vi "PI Ask for Communication Parameters.vi"() -> (10 "Termination character out":T2[](array[typedef])=[enum."LF"], 11 "Syntax out":T1[](array[typedef])=[enum."GCS 1.0"], 12 "TCP/IP Configuration out":T3(array[cluster])=[{"Host address/name"="localhost", "Port"=50000, "Board"=0}], 13 "Flow control out":T6(array[cluster])=[{"input XON/XOFF"=FALSE, "input HW Handshake"=FALSE, "input alt HW HShk"=FALSE, "output XON/XOFF"=FALSE, "output HW Handshake"=FALSE, "output alt HW HShk"=FALSE, "XOFF byte "=19, "XON byte"=17, "parity error byte"=0}] {"parity error byte" format="%.0x"; "XON byte" format="%.0x"; "XOFF byte" format="%.0x"}, 15 "How many\nsystems? out":i32=1 min=1 max=4 step=1, 16 "Abort out":bool=TRUE, 17 "Interface configuration out":T14(array[cluster])=[{"RS232 Portnumber"=0, "Timeout"=1000, "RS232 baud rate"=57600, "Interface"=0, "GPIB Bus"=0, "GPIB address"=4, "GPIB Mode"=0}] {"Interface" items=["RS232", "GPIB", "DLL", "TCP-IP", "USB", "Analog"]; "RS232 Portnumber" items=["COM1", "COM2", "COM3", "COM4", "COM5", "COM6", "COM7", "COM8", "COM9", "COM10", "COM11", "COM12", "COM13", "COM14", "COM15", "COM16", "COM17", "COM18", "COM19", "COM20", "COM21", "COM22", "COM23", "COM24", "COM25", "COM26", "COM27", "COM28", "COM29", "COM30"]}, 18 "DLL Interface\nconfiguration out":T11(array[cluster])=[{"DLL for Device"=0, "DLL Interface"=2, "Parameter"="1"}] {"DLL for Device" items=["C-843", "C-844", "E-710", "C-843.PM", "C-865", "E-761", "Mercury", "E-755", "E-753", "C-866", "E-712", "E-725", "E-861", "C-867", "E-517", "E-816", "E-709", "PI_GCS2_DLL", "HydraPollux"]; "DLL Interface" items=["RS232", "GPIB", "Board", "TCP-IP", "USB", "RS232_DC", "USB_DC", "TCPIP_DC"]})   [LabVIEW 2020]
doc: "A user-interface VI for setting up communications parameters (RS-232 or GPIB, number of systems, baudrate, timeout etc.) for up to 4 systems. Press F1 for displaying a help window with the appropriate interface configuration of each PI controller."
uses:
  Available interfaces.ctl
  Available DLLs.ctl
  Available DLL interfaces.ctl
  Termination character.ctl
  Syntax.ctl
panel:
  in  "Hide help":bool
  in  "Show help":bool
  in  "Help string":string="\nHELP for PI Ask for Communication Parameters.vi\n\nThis VI is a user-interface VI for setting up communications parameters (interface type, number of systems, baudrate, timeout etc.) for up to 4 systems.\nSelect the number of connected systems first. Select the corresponding interface configuration parameters then in the order described below.\n\nPress F10 to return to the VI.\n\nC-413: \tInterface = RS232, DLL, or TCP/IP. TCP/IP support available depending on controller version! If unsure whether your controller supports TCP/IP communication, please refer to the controller user manual), RS232: Input and output HW handshake must be TRUE. DLL: DLL for Device = PI_GCS2_DLL, DLL Interface = USB, Parameter = Serial no. of system to connect to. Syntax: GCS 2.0; Term char = LF.\n\nC-414: \tInterface = RS232, DLL, or TCP/IP. RS232: Input and output HW handshake must be TRUE. DLL: DLL for Device = PI_GCS2_DLL, DLL Interface = USB, Parameter = Serial no. of system to connect to. Syntax: GCS 2.0; Term char = LF.\n\nC-702: \tInterface = RS232 or TCP/IP, RS232: Input and output HW handshake \tmust \tbe TRUE. Syntax: GCS 1.0; Term char = LF.\n\nC-843: \tInterface = DLL, DLL for Device = C-843, DLL Interface = Board, \tParameter = Board number (1 for first C-843 board). Syntax: GCS 1.0; \tTerm char = LF.\n\nC-843.PM: \tInterface = DLL, DLL for Device = C-843.PM, DLL Interface = Board, \tParameter = Board number (1 for first C-843 board). Syntax: GCS 1.0; \tTerm char = LF.\n\nC-865: \tInterface = DLL, DLL for Device = C-865, DLL Interface = RS232, \tParameter = empty string, RS232 baud rate = set as appropriate. Syntax: \tGCS 1.0; Term char = LF.\n\nC-866: \tInterface = DLL, DLL for Device = C-866, DLL Interface = RS232 or USB, \tRS232: Parameter = empty string, RS232 baud rate = set as appropriate, \tUSB: Parameter = Serial no. of system to connect to, \n\tSyntax: GCS 1.0; Term char = LF.\n\nC-867: \tSingle Device: Interface = RS232, TCP/IP or DLL, RS232: Input and output HW \thandshake must be FALSE. DLL (USB): DLL for Device = C-867, DLL \tInterface = USB, Parameter = Serial no. of system to connect to.\nDaisyChain: Interface = DLL, DLL for Device = C-867, DLL Interface = \tRS232_DC, Parameter = Number of device in chain, \tRegister DC: \tFALSE. Syntax: GCS 2.0; Term char = LF.\n\nC-880, C-848: \tInterface = RS232 or GPIB, RS232: Input and output HW handshake must \tbe TRUE. Syntax: GCS 1.0; Term char = LF.\n\nC-880K005: \tInterface = RS232, Input and output HW handshake must be FALSE. \tSyntax: GCS 1.0; Term char = LF.\n\nC-884: \tInterface = RS232, TCP/IP or DLL, RS232: Input and output HW handshake must be FALSE. DLL (USB): DLL for Device = PI_GCS2_DLL, DLL Interface = USB, Parameter = Serial no. of system to connect to. Syntax: GCS 2.0; Term char = LF.\n\nC-885: \tInterface = TCP/IP or DLL. DLL (USB): DLL for Device = PI_GCS2_DLL, DLL Interface = USB, Parameter = Serial no. of system to connect to. Syntax: GCS 2.0; Term char = LF.\nDaisyChain: Interface = DLL, DLL for Device = PI_GCS2_DLL, DLL Interface = \tTCPIP_DC or USB_DC, Parameter = Number of device in chain, \tRegister DC: \tFALSE. Syntax: GCS 2.0; Term char = LF.\n\nC-886: \tInterface = TCP/IP or DLL. DLL (USB): DLL for Device = PI_GCS2_DLL, DLL Interface = USB, Parameter = Serial no. of system to connect to. Syntax: GCS 2.0; Term char = LF.\n\nC-887, F-206, M-8X0: \tFor GCS syntax version = GCS 1.0 (older firmware or compatibility mode, \tcan be set with CSV.vi), Interface = RS232, GPIB (not available for C-887 \tcontroller) or TCP/IP., The error status will not be cleared by this VI. The \tfirst ERR? query will report a hidden error with error code 1, which will be \tcleared during system initialization (INI). RS232: Input and output \thandshake settings must be FALSE. Syntax: GCS 1.0; Term char = \tLF.\nFor GCS syntax version = GCS 2.0 (C-887 Controller), Interface = RS232 \tor TCP/IP. RS232: Input and output handshake settings must be FALSE. \tSyntax: GCS 2.0; Term char = LF.\n\nE-135: Interface = RS232, TCP/IP or DLL: Input and output HW \thandshake must be FALSE. DLL (USB): DLL for Device = \tPI_GCS2_DLL, DLL Interface = USB, Parameter = Serial no. of system to \tconnect to. Syntax: GCS 2.0; Term char = LF.\n\nE-516: \tInterface = RS232 or GPIB, RS232: Input and output HW handshake must \tbe TRUE. Syntax: GCS 1.0; Term char = LF.\n\nE-517: \tInterface = RS232, GPIB, TCP/IP or DLL, RS232: Input and output HW \thandshake must be TRUE, DLL (USB): DLL for Device = E-517, DLL \tInterface = USB, Parameter = Serial no. of system to connect to. Syntax: GCS 2.0; Term char = LF.\n\nE-518: \t\tInterface = RS232, TCP/IP or DLL, RS232: Input and output HW handshake must be TRUE, DLL (USB): DLL for Device = PI_GCS2_DLL, DLL Interface = USB, Parameter = Serial no. of system to connect to. Syntax: GCS 2.0; Term char = LF.\n\nE-709: \tInterface = RS232 or DLL, RS232: Input and output HW handshake \tmust be TRUE. DLL (USB): DLL for Device = E-709, DLL Interface = USB, \tParameter = Serial no. of system to connect to. Syntax: GCS 2.0; Term \tchar = LF.\n\nE-710:\tInterface = DLL, DLL for Device = E-710, DLL Interface = RS232 or GPIB, \tParameter = empty string. Syntax: GCS 1.0; Term char = LF.\n\nE-712: \tInterface = RS232, TCP/IP or DLL, RS232: Input and output HW \thandshake must be TRUE. DLL: DLL for Device = E-712, DLL Interface = \tUSB, \tParameter = Serial no. of system to connect to. \n\tSyntax: GCS 2.0; Term char = LF.\n\nE-725: \tInterface = RS232, TCP/IP or DLL, RS232: Input and output HW \thandshake must be TRUE. DLL: DLL for Device = E-725, DLL Interface = \tUSB, \tParameter = Serial no. of system to connect to. \nSyntax: GCS 2.0; Term char = LF.\n\nE-727: \tInterface = RS232, TCP/IP or DLL, RS232: Input and output HW \thandshake must be TRUE. DLL: DLL for Device = PI_GCS2_DLL, DLL Interface = \tUSB, \tParameter = Serial no. of system to connect to. Syntax: GCS 2.0; Term char = LF.\n\nE-753: \tInterface = RS232 or TCP/IP, RS232: Input and output HW handshake \tmust \tbe TRUE. Syntax: GCS 2.0; Term char = LF.\n\nE-754: Interface = RS232, TCP/IP or DLL, RS232: Input and output HW handshake must be TRUE. DLL: DLL for Device = E-754, DLL Interface = USB, Parameter = Serial no. of system to connect to. Syntax: GCS 2.0; Term char = LF.\n\nE-755:\tSingle Device: Interface = RS232, Input and output HW handshake must \tbe TRUE. DaisyChain: Interface = DLL, DLL for Device = E-755, DLL \tInterface = RS232_DC, Parameter = Number of device in chain (first \tdevice: 1). Syntax: GCS 2.0; Term char = LF.\n\nE-761:\tInterface = DLL, DLL for Device = E-761, DLL Interface = Board, \tParameter = Board number (1 for first E-761 board). Syntax: GCS 1.0; \tTerm char = LF.\n\nE-816: \tInterface = RS232 or DLL, RS232: Input and output HW handshake must \tbe TRUE. DLL (USB): DLL for Device = E-816, DLL Interface = USB, \tParameter = Serial no. of system to connect to. Syntax: GCS 1.0; Term \tchar = LF. \n\nE-861: \tSingle Device: Interface = RS232 or DLL, RS232: Input and output HW \thandshake must be FALSE. DLL (USB): DLL for Device = E-861, DLL \tInterface = USB, Parameter = Serial no. of system to connect to.\nDaisyChain: Interface = DLL, DLL for Device = E-861, DLL Interface = \tRS232_DC or USB_DC, Parameter = Number of device in chain (first device: 1), \tRegister DC: FALSE. Syntax: GCS 2.0; Term char = LF.\n\nE-870: \tInterface = DLL, DLL (USB): DLL for Device = PI_GCS2_DLL, DLL \tInterface = USB, Parameter = Serial no. of system to connect to.\nSyntax: GCS 2.0; Term char = LF.\n\nE-871: Single Device: Interface = RS232 or DLL, RS232: Input and output HW \thandshake must be FALSE. DLL (USB): DLL for Device = \tPI_GCS2_DLL, DLL Interface = USB, Parameter = Serial no. of system to \tconnect to.\nDaisyChain: Interface = DLL, DLL for Device = PI_GCS2_DLL, DLL \tInterface = RS232_DC or USB_DC, Parameter = Number of device in \tchain, Register DC: FALSE. Syntax: GCS 2.0; Term char = LF.\n\nE-872: Interface = RS232, TCP/IP or DLL, RS232: Input and output HW handshake must be FALSE. DLL (USB): DLL for Device = PI_GCS2_DLL, DLL Interface = USB, Parameter = Serial no. of system to \tconnect to.\n\nE-873: Interface = RS232, TCP/IP or DLL, RS232: Input and output HW handshake must be FALSE. DLL (USB): DLL for Device = PI_GCS2_DLL, DLL Interface = USB, Parameter = Serial no. of system to \tconnect to.\n\nE-874: Interface = RS232, TCP/IP or DLL, RS232: Input and output HW handshake must be FALSE. DLL (USB): DLL for Device = PI_GCS2_DLL, DLL Interface = USB, Parameter = Serial no. of system to \tconnect to\n\nHydra: \tInterface = DLL, DLL (TCP/IP and RS-232): DLL for Device = \t\tPI_HydraPollux_GCS2_DLL, DLL Interface = RS232 or TCP/IP, Syntax: \tGCS 2.0; Term char = LF.\n\nMercury™: \tInterface = DLL, DLL for Device = Mercury™, DLL Interface = RS232 \t(even if using USB), Parameter = empty string, RS232 baud rate = same \tas set on controller hardware, Syntax: GCS 1.0; Term char = LF.\n\nGCS_Mercury: \tSingle Device: Interface = RS232 or DLL, RS232: Input and output HW \thandshake must be FALSE. DLL (USB): DLL for Device = PI_GCS2_DLL, \tDLL Interface = USB, Parameter = Serial no. of system to connect to. \tDaisyChain: Interface = DLL, DLL for Device = PI_GCS2_DLL, DLL \tInterface = RS232_DC or USB_DaisyChain, Parameter = Number of device in chain, \tRegister DC: \tFALSE. Syntax: GCS 2.0; Term char = LF.\n\nPollux: \tInterface = DLL, DLL (RS-232): DLL for Device = PI_HydraPollux_GCS2_DLL, DLL Interface = RS232, Baudrate must be 19200, Syntax: GCS 2.0; Term char = LF.\n\n"
  in  "TCP/IP\nConfiguration 2":T4={"Host address/name"="Z-A521-2.pi.ws", "Port"=3000, "Board"=0}
  in  "RS 16":string
  in  "RS 15":string
  in  "RS 14":string
  in  "RS 13":string
  in  "Flow control":T5={"input XON/XOFF"=FALSE, "input HW Handshake"=FALSE, "input alt HW HShk"=FALSE, "output XON/XOFF"=FALSE, "output HW Handshake"=FALSE, "output alt HW HShk"=FALSE, "XOFF byte "=19, "XON byte"=17, "parity error byte"=0} {"parity error byte" format="%.0x"; "XON byte" format="%.0x"; "XOFF byte" format="%.0x"}
  in  "RS 12":string
  in  "RS 11":string
  in  "RS 10":string
  in  "RS 9":string
  in  "RS 8":string
  in  "RS 7":string
  in  "RS 6":string
  in  "RS 5":string
  in  "RS 4":string
  in  "RS 3":string
  in  "RS 2":string
  in  "RS1":string
  in  "DLL Interface\nConfiguration 2":T7 {"DLL Interface" items=["RS232", "GPIB", "Board"]; "DLL for Device" items=["C-843", "C-844"]}
  in  "Interface configuration 2":T8={"RS232 Portnumber"=0, "Timeout"=5000, "RS232 Baud rate"=56000, "Interface"=0, "GPIB Bus"=0, "GPIB Address"=4, "GPIB Mode"=0} {"Interface" items=["RS232", "GPIB", "DLL"]; "RS232 Portnumber" items=["COM1", "COM2", "COM3", "COM4", "COM5", "COM6", "COM7", "COM8", "COM9"]}
  in  "String4":string="System No. 4"
  in  "String3":string="System No. 3"
  in  "String2":string="System No. 2"
  in  "String1":string="System No. 1"
  in  "Interface configuration":T13(array[cluster])=[{"RS232 Portnumber"=0, "Timeout"=1000, "GPIB Bus"=0, "GPIB Address"=4, "GPIB Mode"=0, "DLL for Device"=17, "DLL Interface"=4, "Parameter"="1", "Handshake"=0, "Interface"=0, "Termchar"=enum."LF", "Host address/name"="localhost", "Port"=50000, "Board"=0, "RS232 Baud rate"=4, "Syntax"=enum."GCS 2.0"}, {"RS232 Portnumber"=0, "Timeout"=1000, "GPIB Bus"=0, "GPIB Address"=4, "GPIB Mode"=0, "DLL for Device"=0, "DLL Interface"=2, "Parameter"="1", "Handshake"=0, "Interface"=3, "Termchar"=enum."LF", "Host address/name"="localhost", "Port"=50000, "Board"=0, "RS232 Baud rate"=4, "Syntax"=enum."GCS 1.0"}, {"RS232 Portnumber"=0, "Timeout"=1000, "GPIB Bus"=0, "GPIB Address"=4, "GPIB Mode"=0, "DLL for Device"=0, "DLL Interface"=2, "Parameter"="1", "Handshake"=0, "Interface"=1, "Termchar"=enum."LF", "Host address/name"="localhost", "Port"=50000, "Board"=0, "RS232 Baud rate"=4, "Syntax"=enum."GCS 1.0"}, {"RS232 Portnumber"=0, "Timeout"=1000, "GPIB Bus"=0, "GPIB Address"=4, "GPIB Mode"=0, "DLL for Device"=0, "DLL Interface"=2, "Parameter"="1", "Handshake"=0, "Interface"=2, "Termchar"=enum."LF", "Host address/name"="localhost", "Port"=50000, "Board"=0, "RS232 Baud rate"=4, "Syntax"=enum."GCS 1.0"}] {"RS232 Baud rate" items=["9600", "14400", "19200", "38400", "57600", "115200"]; "Interface" items=["RS232", "GPIB", "DLL", "TCP-IP", "USB", "Analog"]; "Handshake" items=["None", "HW", "XON/XOFF"]; "DLL Interface" items=["RS232", "GPIB", "Board", "TCP-IP", "USB", "RS232_DC", "USB_DC", "TCPIP_DC"]; "DLL for Device" items=["C-843", "C-844", "E-710", "C-843.PM", "C-865", "E-761", "Mercury", "E-755", "E-753", "C-866", "E-712", "E-725", "E-861", "C-867", "E-517", "E-816", "E-709", "PI_GCS2_DLL", "HydraPollux"]; "RS232 Portnumber" items=["COM1", "COM2", "COM3", "COM4", "COM5", "COM6", "COM7", "COM8", "COM9", "COM10", "COM11", "COM12", "COM13", "COM14", "COM15", "COM16", "COM17", "COM18", "COM19", "COM20", "COM21", "COM22", "COM23", "COM24", "COM25", "COM26", "COM27", "COM28", "COM29", "COM30"]}
  in  "Number of systems":i32=1 min=1 max=4 step=1
  in  "abort":bool=TRUE
  in  "ok":bool
  # "Select Interface Parameters"
  # "Interface configuration"
  # "General:"
  # "RS232:"
  # "GPIB:"
  # "DLL:"
  # "TCP/IP:"
  # "TCP/IP:"
  # "TCP/IP:"
  # "DLL:"
  # "General:"
  # "RS232:"
  # "GPIB:"
  # "DLL:"
  # "General:"
  # "RS232:"
  # "GPIB:"
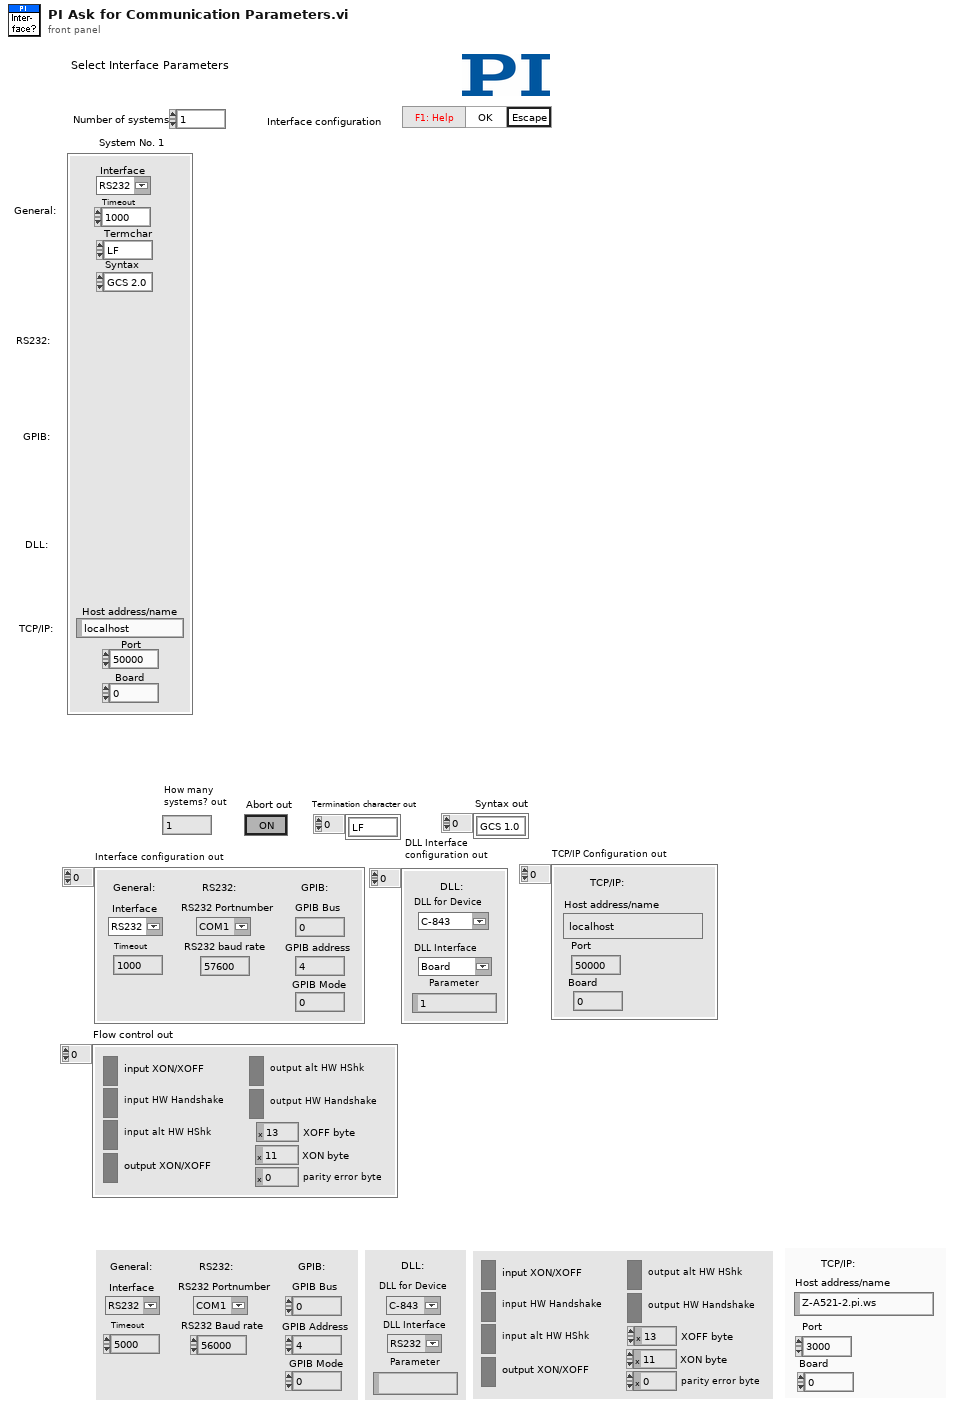
[diagram p1: front panel]
types:
  T1 = typedef "Syntax.ctl" = enum16{"GCS 1.0", "GCS 2.0", "GCS 3.0"}
  T2 = typedef "Termination character.ctl" = enum16{"LF", "CR", "LFCR", "CRLF"}
  T3 = cluster{"Host address/name":string, "Port":i32, "Board":i32}[]
  T4 = cluster{"Host address/name":string, "Port":i32, "Board":i32}
  T5 = cluster{"input XON/XOFF":bool, "input HW Handshake":bool, "input alt HW HShk":bool, "output XON/XOFF":bool, "output HW Handshake":bool, "output alt HW HShk":bool, "XOFF byte ":u8, "XON byte":u8, "parity error byte":u16}
  T6 = cluster{"input XON/XOFF":bool, "input HW Handshake":bool, "input alt HW HShk":bool, "output XON/XOFF":bool, "output HW Handshake":bool, "output alt HW HShk":bool, "XOFF byte ":u8, "XON byte":u8, "parity error byte":u16}[]
  T7 = cluster{"DLL for Device":u16, "DLL Interface":u16, "Parameter":string}
  T8 = cluster{"RS232 Portnumber":u16, "Timeout":u32, "RS232 Baud rate":u32, "Interface":u16, "GPIB Bus":i16, "GPIB Address":i16, "GPIB Mode":i16}
  T9 = typedef "Available DLLs.ctl" = u16
  T10 = typedef "Available DLL interfaces.ctl" = u16
  T11 = cluster{"DLL for Device":T9, "DLL Interface":T10, "Parameter":string}[]
  T12 = typedef "Available interfaces.ctl" = u16
  T13 = cluster{"RS232 Portnumber":u16, "Timeout":i32, "GPIB Bus":i16, "GPIB Address":i16, "GPIB Mode":i16, "DLL for Device":T9, "DLL Interface":T10, "Parameter":string, "Handshake":u16, "Interface":T12, "Termchar":T2, "Host address/name":string, "Port":i32, "Board":i32, "RS232 Baud rate":u16, "Syntax":T1}[]
  T14 = cluster{"RS232 Portnumber":u16, "Timeout":u32, "RS232 baud rate":u32, "Interface":T12, "GPIB Bus":i16, "GPIB address":i16, "GPIB Mode":i16}[]
  T15 = cluster{"input XON/XOFF":bool, "input HW Handshake":bool, "input alt HW HShk":bool, "output XON/XOFF":bool, "output HW Handshake":bool, "output alt HW HShk":bool, "XOFF byte":u8, "XON byte":u8, "parity error byte":u16}[]
  T16 = cluster{"DLL for Device":u16, "DLL Interface":u16, "Parameter":string}[]
  T17 = cluster{"RS232 Portnumber":u16, "Timeout":u32, "RS232 Baud rate":u32, "Interface":T12, "GPIB Bus":i16, "GPIB Address":i16, "GPIB Mode":i16}[]
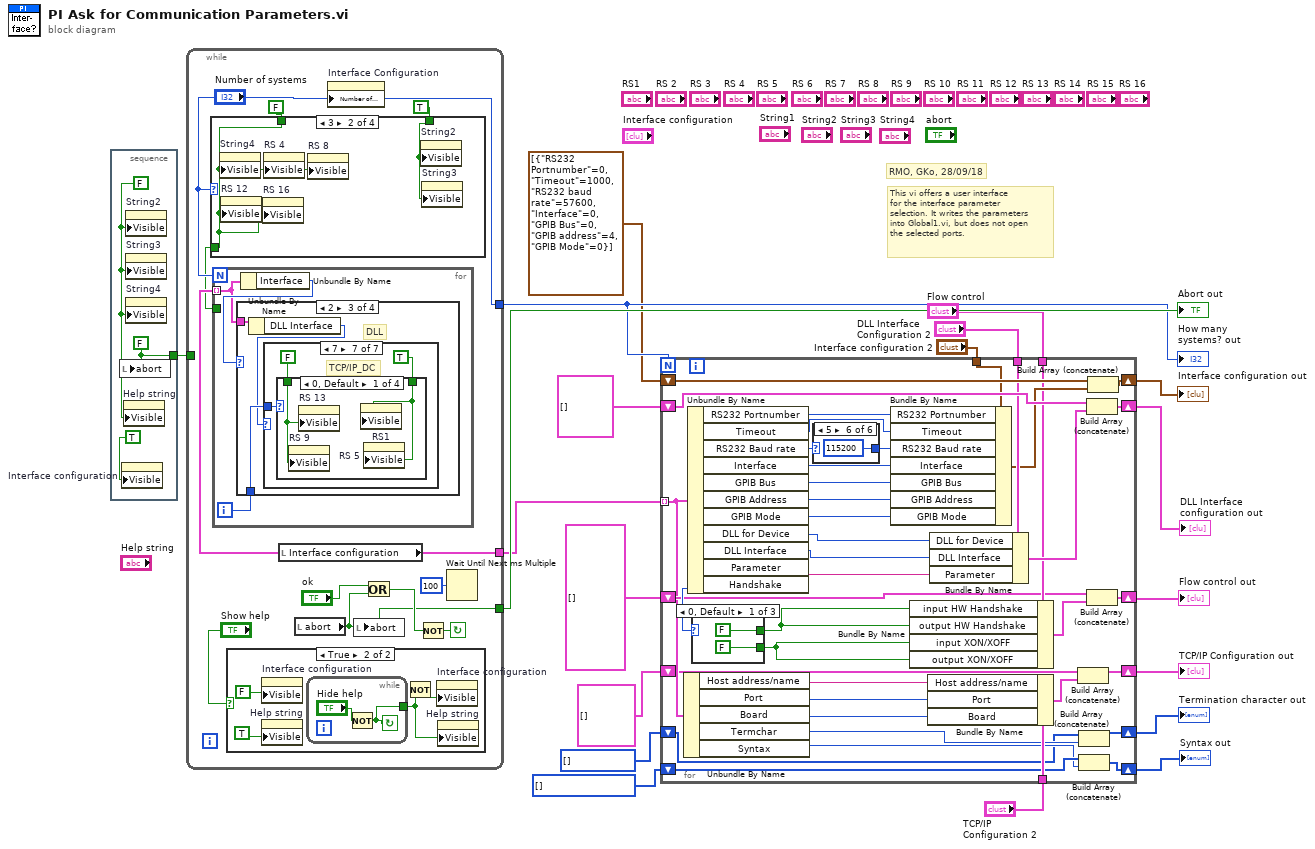
[diagram p0: block diagram]
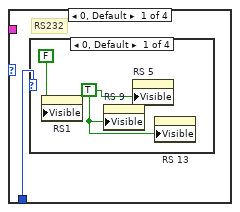
[diagram p3: hidden frame]
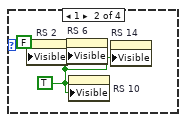
[diagram p4: hidden frame]
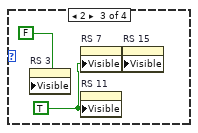
[diagram p5: hidden frame]
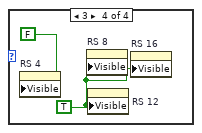
[diagram p6: hidden frame]
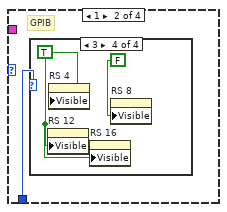
[diagram p7: hidden frame]
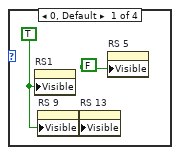
[diagram p8: hidden frame]
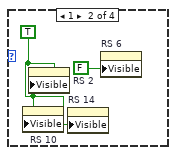
[diagram p9: hidden frame]
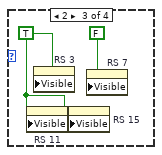
[diagram p10: hidden frame]
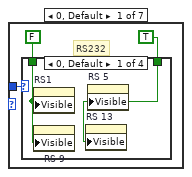
[diagram p11: hidden frame]
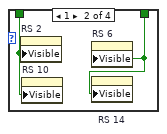
[diagram p12: hidden frame]
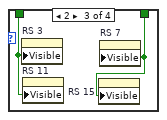
[diagram p13: hidden frame]
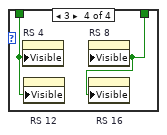
[diagram p14: hidden frame]
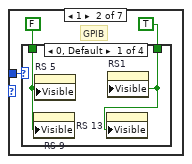
[diagram p15: hidden frame]
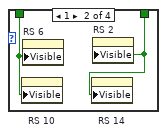
[diagram p16: hidden frame]
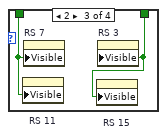
[diagram p17: hidden frame]
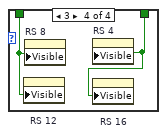
[diagram p18: hidden frame]
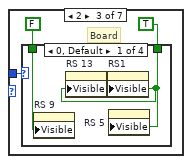
[diagram p19: hidden frame]
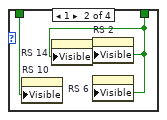
[diagram p20: hidden frame]
diagram:
  w2 = enum16{"GCS 1.0", "GCS 2.0"}[] [] items=["GCS 1.0", "GCS 2.0"]
  w5 = T2[] [] items=["LF", "CR", "LFCR", "CRLF"]
  # "This vi offers a user interface\nfor the interface parameter\nselection. It writes the parameters\ninto Global1.vi, but does not open\nthe selected ports."
  # "RMO, GKo, 28/09/18"
  n1 = stacked-sequence {
    tunnel: [w23] -> w12
    frame #0 {
      w22 = FALSE ("Write Attribute")
      w23 = FALSE
      n2 = local write "abort"(w23) -> ()
      n3 = property on="Interface configuration" class="Arr (strict)"("Visible"=TRUE) -> ()  [unwired: 2 in, 2 out]
      n4 = property on="Help string" class="Str"("Visible"=w22) -> ()  [unwired: 2 in, 2 out]
      n5 = property on="String2" class="Str"("Visible"=w22) -> ()  [unwired: 2 in, 2 out]
      n6 = property on="String3" class="Str"("Visible"=w22) -> ()  [unwired: 2 in, 2 out]
      n7 = property on="String4" class="Str"("Visible"=w22) -> ()  [unwired: 2 in, 2 out]
    }
  }
  n8 = while {
    tunnel: w12 -> [_]
    tunnel: ["Number of systems"] -> w19
    tunnel: [w31] -> w20
    tunnel: [w30] -> w15
    stop <- w33 continue-if-true
    n9 = case shown="3" "Number of systems" {
      tunnel: [w151 w153 w155 w156] -> w27
      tunnel: FALSE ("Write Attribute") -> [w151 w153 _ w156]
      tunnel: TRUE -> [w152 w154 w155 _]
      frame 2 {
        n10 = property on="String3" class="Str"("Visible"=w151) -> ()  [unwired: 2 in, 2 out]
        n11 = property on="String4" class="Str"("Visible"=w151) -> ()  [unwired: 2 in, 2 out]
        n12 = property on="RS 15" class="Str"("Visible"=w151) -> ()  [unwired: 2 in, 2 out]
        n13 = property on="RS 3" class="Str"("Visible"=w151) -> ()  [unwired: 2 in, 2 out]
        n14 = property on="RS 16" class="Str"("Visible"=w151) -> ()  [unwired: 2 in, 2 out]
        n15 = property on="RS 4" class="Str"("Visible"=w151) -> ()  [unwired: 2 in, 2 out]
        n16 = property on="RS 7" class="Str"("Visible"=w151) -> ()  [unwired: 2 in, 2 out]
        n17 = property on="RS 8" class="Str"("Visible"=w151) -> ()  [unwired: 2 in, 2 out]
        n18 = property on="RS 11" class="Str"("Visible"=w151) -> ()  [unwired: 2 in, 2 out]
        n19 = property on="RS 12" class="Str"("Visible"=w151) -> ()  [unwired: 2 in, 2 out]
        n20 = property on="String2" class="Str"("Visible"=w152) -> ()  [unwired: 2 in, 2 out]
      }
      frame 3 {
        n21 = property on="String4" class="Str"("Visible"=w153) -> ()  [unwired: 2 in, 2 out]
        n22 = property on="RS 12" class="Str"("Visible"=w153) -> ()  [unwired: 2 in, 2 out]
        n23 = property on="RS 16" class="Str"("Visible"=w153) -> ()  [unwired: 2 in, 2 out]
        n24 = property on="RS 4" class="Str"("Visible"=w153) -> ()  [unwired: 2 in, 2 out]
        n25 = property on="RS 8" class="Str"("Visible"=w153) -> ()  [unwired: 2 in, 2 out]
        n26 = property on="String2" class="Str"("Visible"=w154) -> ()  [unwired: 2 in, 2 out]
        n27 = property on="String3" class="Str"("Visible"=w154) -> ()  [unwired: 2 in, 2 out]
      }
      frame 4 {
        n28 = property on="String2" class="Str"("Visible"=w155) -> ()  [unwired: 2 in, 2 out]
        n29 = property on="String3" class="Str"("Visible"=w155) -> ()  [unwired: 2 in, 2 out]
        n30 = property on="String4" class="Str"("Visible"=w155) -> ()  [unwired: 2 in, 2 out]
      }
      frame 1, Default {
        n31 = property on="String2" class="Str"("Visible"=w156) -> ()  [unwired: 2 in, 2 out]
        n32 = property on="String3" class="Str"("Visible"=w156) -> ()  [unwired: 2 in, 2 out]
        n33 = property on="String4" class="Str"("Visible"=w156) -> ()  [unwired: 2 in, 2 out]
        n34 = property on="RS 2" class="Str"("Visible"=w156) -> ()  [unwired: 2 in, 2 out]
        n35 = property on="RS 3" class="Str"("Visible"=w156) -> ()  [unwired: 2 in, 2 out]
        n36 = property on="RS 4" class="Str"("Visible"=w156) -> ()  [unwired: 2 in, 2 out]
        n37 = property on="RS 7" class="Str"("Visible"=w156) -> ()  [unwired: 2 in, 2 out]
        n38 = property on="RS 8" class="Str"("Visible"=w156) -> ()  [unwired: 2 in, 2 out]
        n39 = property on="RS 6" class="Str"("Visible"=w156) -> ()  [unwired: 2 in, 2 out]
        n40 = property on="RS 10" class="Str"("Visible"=w156) -> ()  [unwired: 2 in, 2 out]
        n41 = property on="RS 11" class="Str"("Visible"=w156) -> ()  [unwired: 2 in, 2 out]
        n42 = property on="RS 12" class="Str"("Visible"=w156) -> ()  [unwired: 2 in, 2 out]
        n43 = property on="RS 14" class="Str"("Visible"=w156) -> ()  [unwired: 2 in, 2 out]
        n44 = property on="RS 15" class="Str"("Visible"=w156) -> ()  [unwired: 2 in, 2 out]
        n45 = property on="RS 16" class="Str"("Visible"=w156) -> ()  [unwired: 2 in, 2 out]
      }
    }
    n46 = case shown="True" "Show help" {
      frame False {
      }
      frame True {
        n47 = property on="Interface configuration" class="Arr (strict)"("Visible"=FALSE ("Write Attribute")) -> ()  [unwired: 2 in, 2 out]
        n48 = property on="Help string" class="Str"("Visible"=TRUE ("Write Attribute")) -> ()  [unwired: 2 in, 2 out]
        n49 = while {
          tunnel: [w39] -> w36
          stop <- w39 continue-if-true
          n50 = Not(x="Hide help") -> (.not. x?=w39:bool)
        }
        n51 = Not(x=w36) -> (.not. x?=w35:bool)
        n52 = property on="Interface configuration" class="Arr (strict)"("Visible"=w35) -> ()  [unwired: 2 in, 2 out]
        n53 = property on="Help string" class="Str"("Visible"=w36) -> ()  [unwired: 2 in, 2 out]
      }
    }
    n54 = local read "Interface configuration"() -> (w30:T13)
    n55 = for {
      N: "Number of systems" -> [_]
      tunnel: w30 -> [w41] mode=indexing
      tunnel: w27 -> [_]
      i -> [w42]
      n56 = Unbundle By Name(w41) -> ("Interface"=w43:T12)
      n57 = case shown="2" w43 {
        tunnel: w42 -> [w44 w53 w64 w142]
        tunnel: w41 -> [_ _ w63 _]
        frame 0, Default {
          # "RS232"
          n58 = case shown="0, Default" w44 {
            frame 0, Default {
              w45 = TRUE ("Write Attribute")
              n59 = property on="RS1" class="Str"("Visible"=FALSE ("Write Attribute")) -> ()  [unwired: 2 in, 2 out]
              n60 = property on="RS 9" class="Str"("Visible"=w45) -> ()  [unwired: 2 in, 2 out]
              n61 = property on="RS 5" class="Str"("Visible"=w45) -> ()  [unwired: 2 in, 2 out]
              n62 = property on="RS 13" class="Str"("Visible"=w45) -> ()  [unwired: 2 in, 2 out]
            }
            frame 1 {
              w47 = TRUE ("Write Attribute")
              n63 = property on="RS 2" class="Str"("Visible"=FALSE ("Write Attribute")) -> ()  [unwired: 2 in, 2 out]
              n64 = property on="RS 6" class="Str"("Visible"=w47) -> ()  [unwired: 2 in, 2 out]
              n65 = property on="RS 10" class="Str"("Visible"=w47) -> ()  [unwired: 2 in, 2 out]
              n66 = property on="RS 14" class="Str"("Visible"=w47) -> ()  [unwired: 2 in, 2 out]
            }
            frame 2 {
              w49 = TRUE ("Write Attribute")
              n67 = property on="RS 3" class="Str"("Visible"=FALSE ("Write Attribute")) -> ()  [unwired: 2 in, 2 out]
              n68 = property on="RS 7" class="Str"("Visible"=w49) -> ()  [unwired: 2 in, 2 out]
              n69 = property on="RS 11" class="Str"("Visible"=w49) -> ()  [unwired: 2 in, 2 out]
              n70 = property on="RS 15" class="Str"("Visible"=w49) -> ()  [unwired: 2 in, 2 out]
            }
            frame 3 {
              w51 = TRUE ("Write Attribute")
              n71 = property on="RS 4" class="Str"("Visible"=FALSE ("Write Attribute")) -> ()  [unwired: 2 in, 2 out]
              n72 = property on="RS 8" class="Str"("Visible"=w51) -> ()  [unwired: 2 in, 2 out]
              n73 = property on="RS 12" class="Str"("Visible"=w51) -> ()  [unwired: 2 in, 2 out]
              n74 = property on="RS 16" class="Str"("Visible"=w51) -> ()  [unwired: 2 in, 2 out]
            }
          }
        }
        frame 1 {
          # "GPIB"
          n75 = case shown="3" w53 {
            frame 0, Default {
              w54 = TRUE ("Write Attribute")
              n76 = property on="RS1" class="Str"("Visible"=w54) -> ()  [unwired: 2 in, 2 out]
              n77 = property on="RS 9" class="Str"("Visible"=w54) -> ()  [unwired: 2 in, 2 out]
              n78 = property on="RS 13" class="Str"("Visible"=w54) -> ()  [unwired: 2 in, 2 out]
              n79 = property on="RS 5" class="Str"("Visible"=FALSE ("Write Attribute")) -> ()  [unwired: 2 in, 2 out]
            }
            frame 1 {
              w56 = TRUE ("Write Attribute")
              n80 = property on="RS 10" class="Str"("Visible"=w56) -> ()  [unwired: 2 in, 2 out]
              n81 = property on="RS 2" class="Str"("Visible"=w56) -> ()  [unwired: 2 in, 2 out]
              n82 = property on="RS 14" class="Str"("Visible"=w56) -> ()  [unwired: 2 in, 2 out]
              n83 = property on="RS 6" class="Str"("Visible"=FALSE ("Write Attribute")) -> ()  [unwired: 2 in, 2 out]
            }
            frame 2 {
              w58 = TRUE ("Write Attribute")
              n84 = property on="RS 11" class="Str"("Visible"=w58) -> ()  [unwired: 2 in, 2 out]
              n85 = property on="RS 3" class="Str"("Visible"=w58) -> ()  [unwired: 2 in, 2 out]
              n86 = property on="RS 15" class="Str"("Visible"=w58) -> ()  [unwired: 2 in, 2 out]
              n87 = property on="RS 7" class="Str"("Visible"=FALSE ("Write Attribute")) -> ()  [unwired: 2 in, 2 out]
            }
            frame 3 {
              w60 = TRUE ("Write Attribute")
              n88 = property on="RS 12" class="Str"("Visible"=w60) -> ()  [unwired: 2 in, 2 out]
              n89 = property on="RS 4" class="Str"("Visible"=w60) -> ()  [unwired: 2 in, 2 out]
              n90 = property on="RS 16" class="Str"("Visible"=w60) -> ()  [unwired: 2 in, 2 out]
              n91 = property on="RS 8" class="Str"("Visible"=FALSE ("Write Attribute")) -> ()  [unwired: 2 in, 2 out]
            }
          }
        }
        frame 2 {
          # "DLL"
          n92 = Unbundle By Name(w63) -> ("DLL Interface"=w62:T10)
          n93 = case shown="7" w62 {
            tunnel: w64 -> [w67 w78 w89 w100 w111 w122 w133]
            frame 0, Default {
              # "RS232"
              n94 = case shown="0, Default" w67 {
                tunnel: FALSE ("Write Attribute") -> [w69 w71 w73 w75]
                tunnel: TRUE ("Write Attribute") -> [w68 w70 w72 w74]
                frame 0, Default {
                  n95 = property on="RS1" class="Str"("Visible"=w69) -> ()  [unwired: 2 in, 2 out]
                  n96 = property on="RS 9" class="Str"("Visible"=w69) -> ()  [unwired: 2 in, 2 out]
                  n97 = property on="RS 13" class="Str"("Visible"=w68) -> ()  [unwired: 2 in, 2 out]
                  n98 = property on="RS 5" class="Str"("Visible"=w68) -> ()  [unwired: 2 in, 2 out]
                }
                frame 1 {
                  n99 = property on="RS 2" class="Str"("Visible"=w71) -> ()  [unwired: 2 in, 2 out]
                  n100 = property on="RS 10" class="Str"("Visible"=w71) -> ()  [unwired: 2 in, 2 out]
                  n101 = property on="RS 6" class="Str"("Visible"=w70) -> ()  [unwired: 2 in, 2 out]
                  n102 = property on="RS 14" class="Str"("Visible"=w70) -> ()  [unwired: 2 in, 2 out]
                }
                frame 2 {
                  n103 = property on="RS 3" class="Str"("Visible"=w73) -> ()  [unwired: 2 in, 2 out]
                  n104 = property on="RS 11" class="Str"("Visible"=w73) -> ()  [unwired: 2 in, 2 out]
                  n105 = property on="RS 15" class="Str"("Visible"=w72) -> ()  [unwired: 2 in, 2 out]
                  n106 = property on="RS 7" class="Str"("Visible"=w72) -> ()  [unwired: 2 in, 2 out]
                }
                frame 3 {
                  n107 = property on="RS 4" class="Str"("Visible"=w75) -> ()  [unwired: 2 in, 2 out]
                  n108 = property on="RS 12" class="Str"("Visible"=w75) -> ()  [unwired: 2 in, 2 out]
                  n109 = property on="RS 8" class="Str"("Visible"=w74) -> ()  [unwired: 2 in, 2 out]
                  n110 = property on="RS 16" class="Str"("Visible"=w74) -> ()  [unwired: 2 in, 2 out]
                }
              }
            }
            frame 1 {
              # "GPIB"
              n111 = case shown="0, Default" w78 {
                tunnel: FALSE ("Write Attribute") -> [w80 w82 w84 w86]
                tunnel: TRUE ("Write Attribute") -> [w79 w81 w83 w85]
                frame 0, Default {
                  n112 = property on="RS 9" class="Str"("Visible"=w80) -> ()  [unwired: 2 in, 2 out]
                  n113 = property on="RS 5" class="Str"("Visible"=w80) -> ()  [unwired: 2 in, 2 out]
                  n114 = property on="RS 13" class="Str"("Visible"=w79) -> ()  [unwired: 2 in, 2 out]
                  n115 = property on="RS1" class="Str"("Visible"=w79) -> ()  [unwired: 2 in, 2 out]
                }
                frame 1 {
                  n116 = property on="RS 10" class="Str"("Visible"=w82) -> ()  [unwired: 2 in, 2 out]
                  n117 = property on="RS 6" class="Str"("Visible"=w82) -> ()  [unwired: 2 in, 2 out]
                  n118 = property on="RS 14" class="Str"("Visible"=w81) -> ()  [unwired: 2 in, 2 out]
                  n119 = property on="RS 2" class="Str"("Visible"=w81) -> ()  [unwired: 2 in, 2 out]
                }
                frame 2 {
                  n120 = property on="RS 11" class="Str"("Visible"=w84) -> ()  [unwired: 2 in, 2 out]
                  n121 = property on="RS 7" class="Str"("Visible"=w84) -> ()  [unwired: 2 in, 2 out]
                  n122 = property on="RS 15" class="Str"("Visible"=w83) -> ()  [unwired: 2 in, 2 out]
                  n123 = property on="RS 3" class="Str"("Visible"=w83) -> ()  [unwired: 2 in, 2 out]
                }
                frame 3 {
                  n124 = property on="RS 12" class="Str"("Visible"=w86) -> ()  [unwired: 2 in, 2 out]
                  n125 = property on="RS 8" class="Str"("Visible"=w86) -> ()  [unwired: 2 in, 2 out]
                  n126 = property on="RS 4" class="Str"("Visible"=w85) -> ()  [unwired: 2 in, 2 out]
                  n127 = property on="RS 16" class="Str"("Visible"=w85) -> ()  [unwired: 2 in, 2 out]
                }
              }
            }
            frame 2 {
              # "Board"
              n128 = case shown="0, Default" w89 {
                tunnel: FALSE ("Write Attribute") -> [w91 w93 w95 w97]
                tunnel: TRUE ("Write Attribute") -> [w90 w92 w94 w96]
                frame 0, Default {
                  n129 = property on="RS 9" class="Str"("Visible"=w91) -> ()  [unwired: 2 in, 2 out]
                  n130 = property on="RS 13" class="Str"("Visible"=w90) -> ()  [unwired: 2 in, 2 out]
                  n131 = property on="RS1" class="Str"("Visible"=w90) -> ()  [unwired: 2 in, 2 out]
                  n132 = property on="RS 5" class="Str"("Visible"=w90) -> ()  [unwired: 2 in, 2 out]
                }
                frame 1 {
                  n133 = property on="RS 10" class="Str"("Visible"=w93) -> ()  [unwired: 2 in, 2 out]
                  n134 = property on="RS 14" class="Str"("Visible"=w92) -> ()  [unwired: 2 in, 2 out]
                  n135 = property on="RS 2" class="Str"("Visible"=w92) -> ()  [unwired: 2 in, 2 out]
                  n136 = property on="RS 6" class="Str"("Visible"=w92) -> ()  [unwired: 2 in, 2 out]
                }
                frame 2 {
                  n137 = property on="RS 11" class="Str"("Visible"=w95) -> ()  [unwired: 2 in, 2 out]
                  n138 = property on="RS 15" class="Str"("Visible"=w94) -> ()  [unwired: 2 in, 2 out]
                  n139 = property on="RS 3" class="Str"("Visible"=w94) -> ()  [unwired: 2 in, 2 out]
                  n140 = property on="RS 7" class="Str"("Visible"=w94) -> ()  [unwired: 2 in, 2 out]
                }
                frame 3 {
                  n141 = property on="RS 12" class="Str"("Visible"=w97) -> ()  [unwired: 2 in, 2 out]
                  n142 = property on="RS 16" class="Str"("Visible"=w96) -> ()  [unwired: 2 in, 2 out]
                  n143 = property on="RS 4" class="Str"("Visible"=w96) -> ()  [unwired: 2 in, 2 out]
                  n144 = property on="RS 8" class="Str"("Visible"=w96) -> ()  [unwired: 2 in, 2 out]
                }
              }
            }
            frame 4 {
              # "USB"
              n145 = case shown="0, Default" w100 {
                tunnel: FALSE ("Write Attribute") -> [w102 w104 w106 w108]
                tunnel: TRUE ("Write Attribute") -> [w101 w103 w105 w107]
                frame 0, Default {
                  n146 = property on="RS 9" class="Str"("Visible"=w102) -> ()  [unwired: 2 in, 2 out]
                  n147 = property on="RS 13" class="Str"("Visible"=w101) -> ()  [unwired: 2 in, 2 out]
                  n148 = property on="RS1" class="Str"("Visible"=w101) -> ()  [unwired: 2 in, 2 out]
                  n149 = property on="RS 5" class="Str"("Visible"=w101) -> ()  [unwired: 2 in, 2 out]
                }
                frame 1 {
                  n150 = property on="RS 10" class="Str"("Visible"=w104) -> ()  [unwired: 2 in, 2 out]
                  n151 = property on="RS 14" class="Str"("Visible"=w103) -> ()  [unwired: 2 in, 2 out]
                  n152 = property on="RS 2" class="Str"("Visible"=w103) -> ()  [unwired: 2 in, 2 out]
                  n153 = property on="RS 6" class="Str"("Visible"=w103) -> ()  [unwired: 2 in, 2 out]
                }
                frame 2 {
                  n154 = property on="RS 11" class="Str"("Visible"=w106) -> ()  [unwired: 2 in, 2 out]
                  n155 = property on="RS 15" class="Str"("Visible"=w105) -> ()  [unwired: 2 in, 2 out]
                  n156 = property on="RS 3" class="Str"("Visible"=w105) -> ()  [unwired: 2 in, 2 out]
                  n157 = property on="RS 7" class="Str"("Visible"=w105) -> ()  [unwired: 2 in, 2 out]
                }
                frame 3 {
                  n158 = property on="RS 12" class="Str"("Visible"=w108) -> ()  [unwired: 2 in, 2 out]
                  n159 = property on="RS 16" class="Str"("Visible"=w107) -> ()  [unwired: 2 in, 2 out]
                  n160 = property on="RS 4" class="Str"("Visible"=w107) -> ()  [unwired: 2 in, 2 out]
                  n161 = property on="RS 8" class="Str"("Visible"=w107) -> ()  [unwired: 2 in, 2 out]
                }
              }
            }
            frame 5 {
              # "RS232_DC"
              n162 = case shown="1" w111 {
                tunnel: FALSE ("Write Attribute") -> [w112 w114 w116 w118]
                tunnel: TRUE ("Write Attribute") -> [w113 w115 w117 w119]
                frame 0, Default {
                  n163 = property on="RS 9" class="Str"("Visible"=w112) -> ()  [unwired: 2 in, 2 out]
                  n164 = property on="RS 13" class="Str"("Visible"=w113) -> ()  [unwired: 2 in, 2 out]
                  n165 = property on="RS1" class="Str"("Visible"=w112) -> ()  [unwired: 2 in, 2 out]
                  n166 = property on="RS 5" class="Str"("Visible"=w113) -> ()  [unwired: 2 in, 2 out]
                }
                frame 1 {
                  n167 = property on="RS 10" class="Str"("Visible"=w114) -> ()  [unwired: 2 in, 2 out]
                  n168 = property on="RS 14" class="Str"("Visible"=w115) -> ()  [unwired: 2 in, 2 out]
                  n169 = property on="RS 2" class="Str"("Visible"=w114) -> ()  [unwired: 2 in, 2 out]
                  n170 = property on="RS 6" class="Str"("Visible"=w115) -> ()  [unwired: 2 in, 2 out]
                }
                frame 2 {
                  n171 = property on="RS 11" class="Str"("Visible"=w116) -> ()  [unwired: 2 in, 2 out]
                  n172 = property on="RS 15" class="Str"("Visible"=w117) -> ()  [unwired: 2 in, 2 out]
                  n173 = property on="RS 3" class="Str"("Visible"=w116) -> ()  [unwired: 2 in, 2 out]
                  n174 = property on="RS 7" class="Str"("Visible"=w117) -> ()  [unwired: 2 in, 2 out]
                }
                frame 3 {
                  n175 = property on="RS 12" class="Str"("Visible"=w118) -> ()  [unwired: 2 in, 2 out]
                  n176 = property on="RS 16" class="Str"("Visible"=w119) -> ()  [unwired: 2 in, 2 out]
                  n177 = property on="RS 4" class="Str"("Visible"=w118) -> ()  [unwired: 2 in, 2 out]
                  n178 = property on="RS 8" class="Str"("Visible"=w119) -> ()  [unwired: 2 in, 2 out]
                }
              }
            }
            frame 3 {
              # "TCP/IP"
              n179 = case shown="0, Default" w122 {
                tunnel: FALSE ("Write Attribute") -> [w123 w125 w127 w129]
                tunnel: TRUE ("Write Attribute") -> [w124 w126 w128 w130]
                frame 0, Default {
                  n180 = property on="RS 9" class="Str"("Visible"=w123) -> ()  [unwired: 2 in, 2 out]
                  n181 = property on="RS 13" class="Str"("Visible"=w123) -> ()  [unwired: 2 in, 2 out]
                  n182 = property on="RS1" class="Str"("Visible"=w124) -> ()  [unwired: 2 in, 2 out]
                  n183 = property on="RS 5" class="Str"("Visible"=w124) -> ()  [unwired: 2 in, 2 out]
                }
                frame 1 {
                  n184 = property on="RS 10" class="Str"("Visible"=w125) -> ()  [unwired: 2 in, 2 out]
                  n185 = property on="RS 14" class="Str"("Visible"=w125) -> ()  [unwired: 2 in, 2 out]
                  n186 = property on="RS 2" class="Str"("Visible"=w126) -> ()  [unwired: 2 in, 2 out]
                  n187 = property on="RS 6" class="Str"("Visible"=w126) -> ()  [unwired: 2 in, 2 out]
                }
                frame 2 {
                  n188 = property on="RS 11" class="Str"("Visible"=w127) -> ()  [unwired: 2 in, 2 out]
                  n189 = property on="RS 15" class="Str"("Visible"=w127) -> ()  [unwired: 2 in, 2 out]
                  n190 = property on="RS 3" class="Str"("Visible"=w128) -> ()  [unwired: 2 in, 2 out]
                  n191 = property on="RS 7" class="Str"("Visible"=w128) -> ()  [unwired: 2 in, 2 out]
                }
                frame 3 {
                  n192 = property on="RS 12" class="Str"("Visible"=w129) -> ()  [unwired: 2 in, 2 out]
                  n193 = property on="RS 16" class="Str"("Visible"=w129) -> ()  [unwired: 2 in, 2 out]
                  n194 = property on="RS 4" class="Str"("Visible"=w130) -> ()  [unwired: 2 in, 2 out]
                  n195 = property on="RS 8" class="Str"("Visible"=w130) -> ()  [unwired: 2 in, 2 out]
                }
              }
            }
            frame 7 {
              # "TCP/IP_DC"
              n196 = case shown="0, Default" w133 {
                tunnel: FALSE ("Write Attribute") -> [w135 w136 w138 w140]
                tunnel: TRUE ("Write Attribute") -> [w134 w137 w139 w141]
                frame 0, Default {
                  n197 = property on="RS 9" class="Str"("Visible"=w135) -> ()  [unwired: 2 in, 2 out]
                  n198 = property on="RS 13" class="Str"("Visible"=w135) -> ()  [unwired: 2 in, 2 out]
                  n199 = property on="RS1" class="Str"("Visible"=w134) -> ()  [unwired: 2 in, 2 out]
                  n200 = property on="RS 5" class="Str"("Visible"=w134) -> ()  [unwired: 2 in, 2 out]
                }
                frame 1 {
                  n201 = property on="RS 10" class="Str"("Visible"=w136) -> ()  [unwired: 2 in, 2 out]
                  n202 = property on="RS 14" class="Str"("Visible"=w136) -> ()  [unwired: 2 in, 2 out]
                  n203 = property on="RS 2" class="Str"("Visible"=w137) -> ()  [unwired: 2 in, 2 out]
                  n204 = property on="RS 6" class="Str"("Visible"=w137) -> ()  [unwired: 2 in, 2 out]
                }
                frame 2 {
                  n205 = property on="RS 11" class="Str"("Visible"=w138) -> ()  [unwired: 2 in, 2 out]
                  n206 = property on="RS 15" class="Str"("Visible"=w138) -> ()  [unwired: 2 in, 2 out]
                  n207 = property on="RS 3" class="Str"("Visible"=w139) -> ()  [unwired: 2 in, 2 out]
                  n208 = property on="RS 7" class="Str"("Visible"=w139) -> ()  [unwired: 2 in, 2 out]
                }
                frame 3 {
                  n209 = property on="RS 12" class="Str"("Visible"=w140) -> ()  [unwired: 2 in, 2 out]
                  n210 = property on="RS 16" class="Str"("Visible"=w140) -> ()  [unwired: 2 in, 2 out]
                  n211 = property on="RS 4" class="Str"("Visible"=w141) -> ()  [unwired: 2 in, 2 out]
                  n212 = property on="RS 8" class="Str"("Visible"=w141) -> ()  [unwired: 2 in, 2 out]
                }
              }
            }
          }
        }
        frame 3 {
          # "TCPIP"
          n213 = case shown="0, Default" w142 {
            frame 0, Default {
              w143 = TRUE ("Write Attribute")
              n214 = property on="RS1" class="Str"("Visible"=w143) -> ()  [unwired: 2 in, 2 out]
              n215 = property on="RS 9" class="Str"("Visible"=w143) -> ()  [unwired: 2 in, 2 out]
              n216 = property on="RS 5" class="Str"("Visible"=w143) -> ()  [unwired: 2 in, 2 out]
              n217 = property on="RS 13" class="Str"("Visible"=FALSE ("Write Attribute")) -> ()  [unwired: 2 in, 2 out]
            }
            frame 1 {
              w145 = TRUE ("Write Attribute")
              n218 = property on="RS 10" class="Str"("Visible"=w145) -> ()  [unwired: 2 in, 2 out]
              n219 = property on="RS 2" class="Str"("Visible"=w145) -> ()  [unwired: 2 in, 2 out]
              n220 = property on="RS 6" class="Str"("Visible"=w145) -> ()  [unwired: 2 in, 2 out]
              n221 = property on="RS 14" class="Str"("Visible"=FALSE ("Write Attribute")) -> ()  [unwired: 2 in, 2 out]
            }
            frame 2 {
              w147 = TRUE ("Write Attribute")
              n222 = property on="RS 11" class="Str"("Visible"=w147) -> ()  [unwired: 2 in, 2 out]
              n223 = property on="RS 3" class="Str"("Visible"=w147) -> ()  [unwired: 2 in, 2 out]
              n224 = property on="RS 7" class="Str"("Visible"=w147) -> ()  [unwired: 2 in, 2 out]
              n225 = property on="RS 15" class="Str"("Visible"=FALSE ("Write Attribute")) -> ()  [unwired: 2 in, 2 out]
            }
            frame 3 {
              w149 = TRUE ("Write Attribute")
              n226 = property on="RS 12" class="Str"("Visible"=w149) -> ()  [unwired: 2 in, 2 out]
              n227 = property on="RS 4" class="Str"("Visible"=w149) -> ()  [unwired: 2 in, 2 out]
              n228 = property on="RS 8" class="Str"("Visible"=w149) -> ()  [unwired: 2 in, 2 out]
              n229 = property on="RS 16" class="Str"("Visible"=FALSE ("Write Attribute")) -> ()  [unwired: 2 in, 2 out]
            }
          }
        }
      }
    }
    n230 = local read "abort"() -> (w31:bool)
    n231 = property on="Interface Configuration" class="Arr (strict)"("Number of Columns"="Number of systems") -> ()  [unwired: 2 in, 2 out]
    n232 = local write "abort"(w31) -> ()
    n233 = Or(x="ok", y=w31) -> (x .or. y?=w32:bool)
    n234 = Not(x=w32) -> (.not. x?=w33:bool)
    n235 = Wait Until Next ms Multiple(millisecond multiple=u32 100) -> ()  [unwired: 1 out]
  }
  "Abort out" <- w20
  "How many\nsystems? out" <- w19
  n236 = for {
    N: w19 -> [_]
    tunnel: w15 -> [w173] mode=indexing
    shift-right: [w169] -> w18
    shift-left: T14 [{"RS232 Portnumber"=0, "Timeout"=1000, "RS232 baud rate"=57600, "Interface"=0, "GPIB Bus"=0, "GPIB address"=4, "GPIB Mode"=0}] ("Interface configuration out") -> [w188]
    shift-right: [w185] -> w17
    shift-left: T16 [] -> [w186]
    tunnel: "DLL Interface\nConfiguration 2" -> [w184]
    tunnel: "Interface configuration 2" -> [w182]
    tunnel: "Flow control" -> [w181]
    shift-right: [w177] -> w7
    shift-left: T15 [] -> [w176]
    tunnel: "TCP/IP\nConfiguration 2" -> [w174]
    shift-right: [w168] -> w8
    shift-left: T3 [] -> [w166]
    shift-right: [w164] -> w4
    shift-left: w5 -> [w157]
    shift-right: [w161] -> w3
    shift-left: w2 -> [w160]
    n237 = Unbundle By Name(w173) -> ("Host address/name"=w172:string, "Port"=w171:i32, "Board"=w170:i32, "Termchar"=w165:T2, "Syntax"=w159:T1)
    n238 = Unbundle By Name(w173) -> ("RS232 Portnumber"=w196:u16, "Timeout"=w158:i32, "RS232 Baud rate"=w163:u16, "Interface"=w195:T12, "GPIB Bus"=w194:i16, "GPIB Address"=w193:i16, "GPIB Mode"=w192:i16, "DLL for Device"=w191:T9, "DLL Interface"=w190:T10, "Parameter"=w189:string, "Handshake"=w180:u16)
    n239 = case shown="0, Default" w180 {
      tunnel: [FALSE TRUE FALSE] -> w179
      tunnel: [FALSE FALSE TRUE] -> w178
      frame 0, Default {
      }
      frame 1 {
      }
      frame 2 {
      }
    }
    n240 = case shown="5" w163 {
      tunnel: [9600 14400 19200 38400 57600 115200] -> w162
      frame 0, Default {
      }
      frame 1 {
      }
      frame 2 {
      }
      frame 3 {
      }
      frame 4 {
      }
      frame 5 {
      }
    }
    n241 = Bundle By Name(cluster=w182, "RS232 Portnumber"=w196, "Timeout"=w158, "RS232 Baud rate"=w162, "Interface"=w195, "GPIB Bus"=w194, "GPIB Address"=w193, "GPIB Mode"=w192) -> (w183:T8)
    n242 = Bundle By Name(cluster=w181, "input HW Handshake"=w179, "output HW Handshake"=w179, "input XON/XOFF"=w178, "output XON/XOFF"=w178) -> (w175:T5)
    n243 = Bundle By Name(cluster=w174, "Host address/name"=w172, "Port"=w171, "Board"=w170) -> (w167:T4)
    n244 = Bundle By Name(cluster=w184, "DLL for Device"=w191, "DLL Interface"=w190, "Parameter"=w189) -> (w187:T7)
    n245 = Build Array (concatenate)(w166, w167) -> (w168:T3)
    n246 = Build Array (concatenate)(w157, w165) -> (w164:T2[])
    n247 = Build Array (concatenate)(w160, w159) -> (w161:T1[])
    n248 = Build Array (concatenate)(w186, w187) -> (w185:T16)
    n249 = Build Array (concatenate)(w176, w175) -> (w177:T6)
    n250 = Build Array (concatenate)(w188, w183) -> (w169:T17)
  }
  "Interface configuration out" <- w18
  "DLL Interface\nconfiguration out" <- w17
  "Flow control out" <- w7
  "Termination character out" <- w4
  "TCP/IP Configuration out" <- w8
  "Syntax out" <- w3
